vi "Is SSE Request.vi"(11 "Request in":refnum<class "Request.lvclass">) -> (0 "error out":errorcluster, 2 "Is SSE Request":bool)   [LabVIEW 2020, in "HTTP Server.lvlib" / "SSE Handler.lvclass"]
uses:
  SSE Handler.lvclass
  SSE Handler.lvclass/SSE Handler.ctl
  lv-http-util/HTTP Utils/Request/Request.lvclass
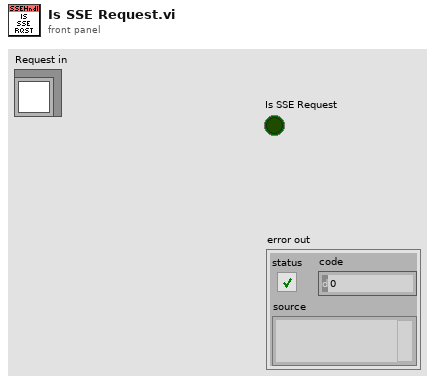
[diagram p1: front panel]
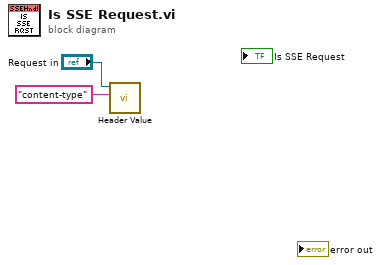
[diagram p0: block diagram]
diagram:
  n1 = call "Header Value.vi"("Header"="content-type", "Request in"="Request in") -> ()  [unwired: 6 in, 4 out]
